vi "Default_V1_1_0_0.vi"() -> (3 "State":T1)   [LabVIEW 2012, in "ListBox_XControl.xctl"]
doc: "Passes out the default state for XControl version 1.1.0.0"
uses:
  ListBox_XControl.xctl
  ListBox_State_1_1_0_0.ctl
  VIs/Order Type Def.ctl
  VIs/Value Filters.ctl
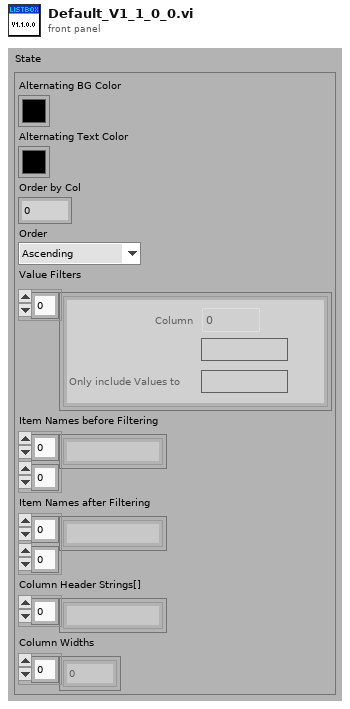
[diagram p1: front panel]
types:
  T1 = typedef "ListBox_XControl.xctl/ListBox_State_1_1_0_0.ctl" = cluster{"Alternating BG Color":u32, "Alternating Text Color":u32, "Order by Col":i32, "Order":T2, "Value Filters":T3, "Item Names before Filtering":string[][], "Item Names after Filtering":string[][], "Column Header Strings[]":string[], "Column Widths":u32[]}
  T2 = typedef "ListBox_XControl.xctl/Order Type Def.ctl" = enum16{"Ascending", "Descending", "Off"}
  T3 = typedef "ListBox_XControl.xctl/Value Filters.ctl" = cluster{"Column":i32, "Only include Values From":string, "Only include Values to":string}[]
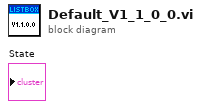
[diagram p0: block diagram]
diagram:
